vi "Write Write Data.vi"(10 "WriteData":bool, 11 "Template in":refnum<class "Template.lvclass">) -> (3 "Template out":refnum<class "Template.lvclass">)   [LabVIEW 2020, in "Template.lvlib" / "Template.lvclass"]
doc: "Sets the Write Data? boolean flag"
uses:
  Template.lvclass
  Template.lvclass/Template.ctl
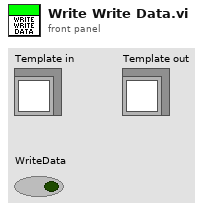
[diagram p1: front panel]
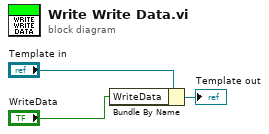
[diagram p0: block diagram]
diagram:
  n1 = Bundle By Name(cluster="Template in", "WriteData"="WriteData") -> (→"Template out":refnum<class "Template.lvclass">)
